vi "NI VeriStand - System Definition File Path.vi"(8 "error in (no error)":errorcluster) -> (0 "error out":errorcluster, 3 "SDF path":path)   [LabVIEW 2020, in "Custom Device Utility Library.lvlib"]
doc: "Returns the file path to the active NI VeriStand system definition file (.nivssdf) after the system definition is deployed."
uses:
  <vilib>/NI VeriStand/Custom Device Tools/Custom Device Utility Library/Custom Device Utility Library.lvlib
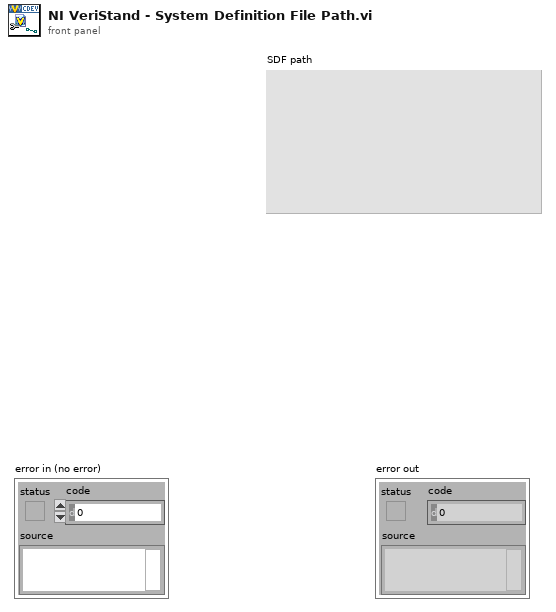
[diagram p1: front panel]
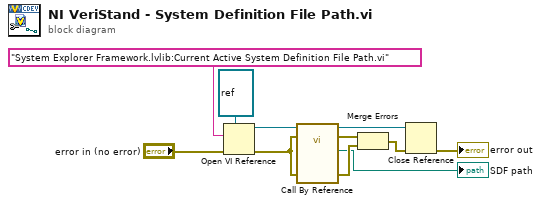
[diagram p0: block diagram]
diagram:
  n1 = Open VI Reference(type specifier VI Refnum (for type only)=refnum<vi> refnum, vi path="System Explorer Framework.lvlib:Current Active System Definition File Path.vi", error in (no error)="error in (no error)") -> (vi reference=w9:refnum<vi>, error out=w7:errorcluster)  [unwired: 3 in]
  n2 = call-by-ref "?"(reference=w9, error in=w7, 8:"error in (no error)"=w7) -> (reference out=w3:refnum<vi>, error out=w6:errorcluster, 0:"error out"=w5:errorcluster, "Active System Definition Path"=→"SDF path":path)  [unwired: 9 in]
  n3 = Merge Errors(w6, w5) -> (w4:errorcluster)
  n4 = Close Reference(reference=w3, error in (no error)=w4) -> (error out=→"error out":errorcluster)
